vi "运维调试_CODCr.vi"() -> ()   [LabVIEW 2016, in "CODCr库.lvlib"]
uses:
  <vilib>/Utility/miscctls.llb/LVPointTypeDef.ctl
  <vilib>/Plasmionique/MB Master/MB_Master_Serial/MB_Master_Serial.lvclass
  D:/Program Files (x86)/National Instruments/LabVIEW 2016/vi.lib/Plasmionique/MB Master/MB_Master/MB_Master.lvclass
  <vilib>/Plasmionique/MB Master/MB Master.lvlib
  <vilib>/ptbypt/NI_PtbyPt.lvlib
panel:
  out "COM口":string
  in  "空白测试":bool
  in  "隐藏按钮":bool
  in  "写入消解温度时长":bool
  in  "保存KB值":bool
  out "source":string
  in  "标样核查":bool
  out "启动时间":timestamp format="%<%Y/%m/%d %H:%M:%S>T"
  out "主循环次数":i32
  out "status":bool
  out "启动测量模式":T1(ring)
  out "曲线斜率B":sgl format="%#_10g"
  out "曲线斜率K":sgl format="%#_10g"
  out "量程上限":sgl
  out "量程下限":sgl
  out "消解时长":u16
  out "消解温度":u16
  out "测量精度":u16
  out "测量结果":sgl
  out "标样参考值":sgl
  out "量程":u16
  out "工作状态":T1(ring)
  out "仪器时间":timestamp format="%<%X\n%x>T"
  out "关键参数区":T2
  out "状态告警区":T3
  out "测量数据区":T4 {"单位" items=["ug/L", "mg/L", "ppm", "mg/m3", "cm", "ppb", "ug/m3", "%", "nmol/mol", "umol/mol", "MPN/L", "MPN/100ml", "ng/m3", "NTU", "无量纲", "ms/cm", "us/cm", "℃", "mV", "万个/L"]}
  out "系统时间":timestamp format="%<%Y/%m/%d %H:%M:%S>T"
  in  "VISA Resource":refnum<visa-resource-name>="COM9"
  out "Registers":u16[](array[numeric])
  in  "枚举":enum16{"读取", "写入", "读取参数"}(ring)
  in  "停止":bool
  in  "校时":bool
  in  "标样校准":bool
  in  "空白校准":bool
  in  "零点核查":bool
  in  "跨度核查":bool
  in  "水样测试":bool
  in  "返回":bool
  in  "设置":bool
  # "mg/L"
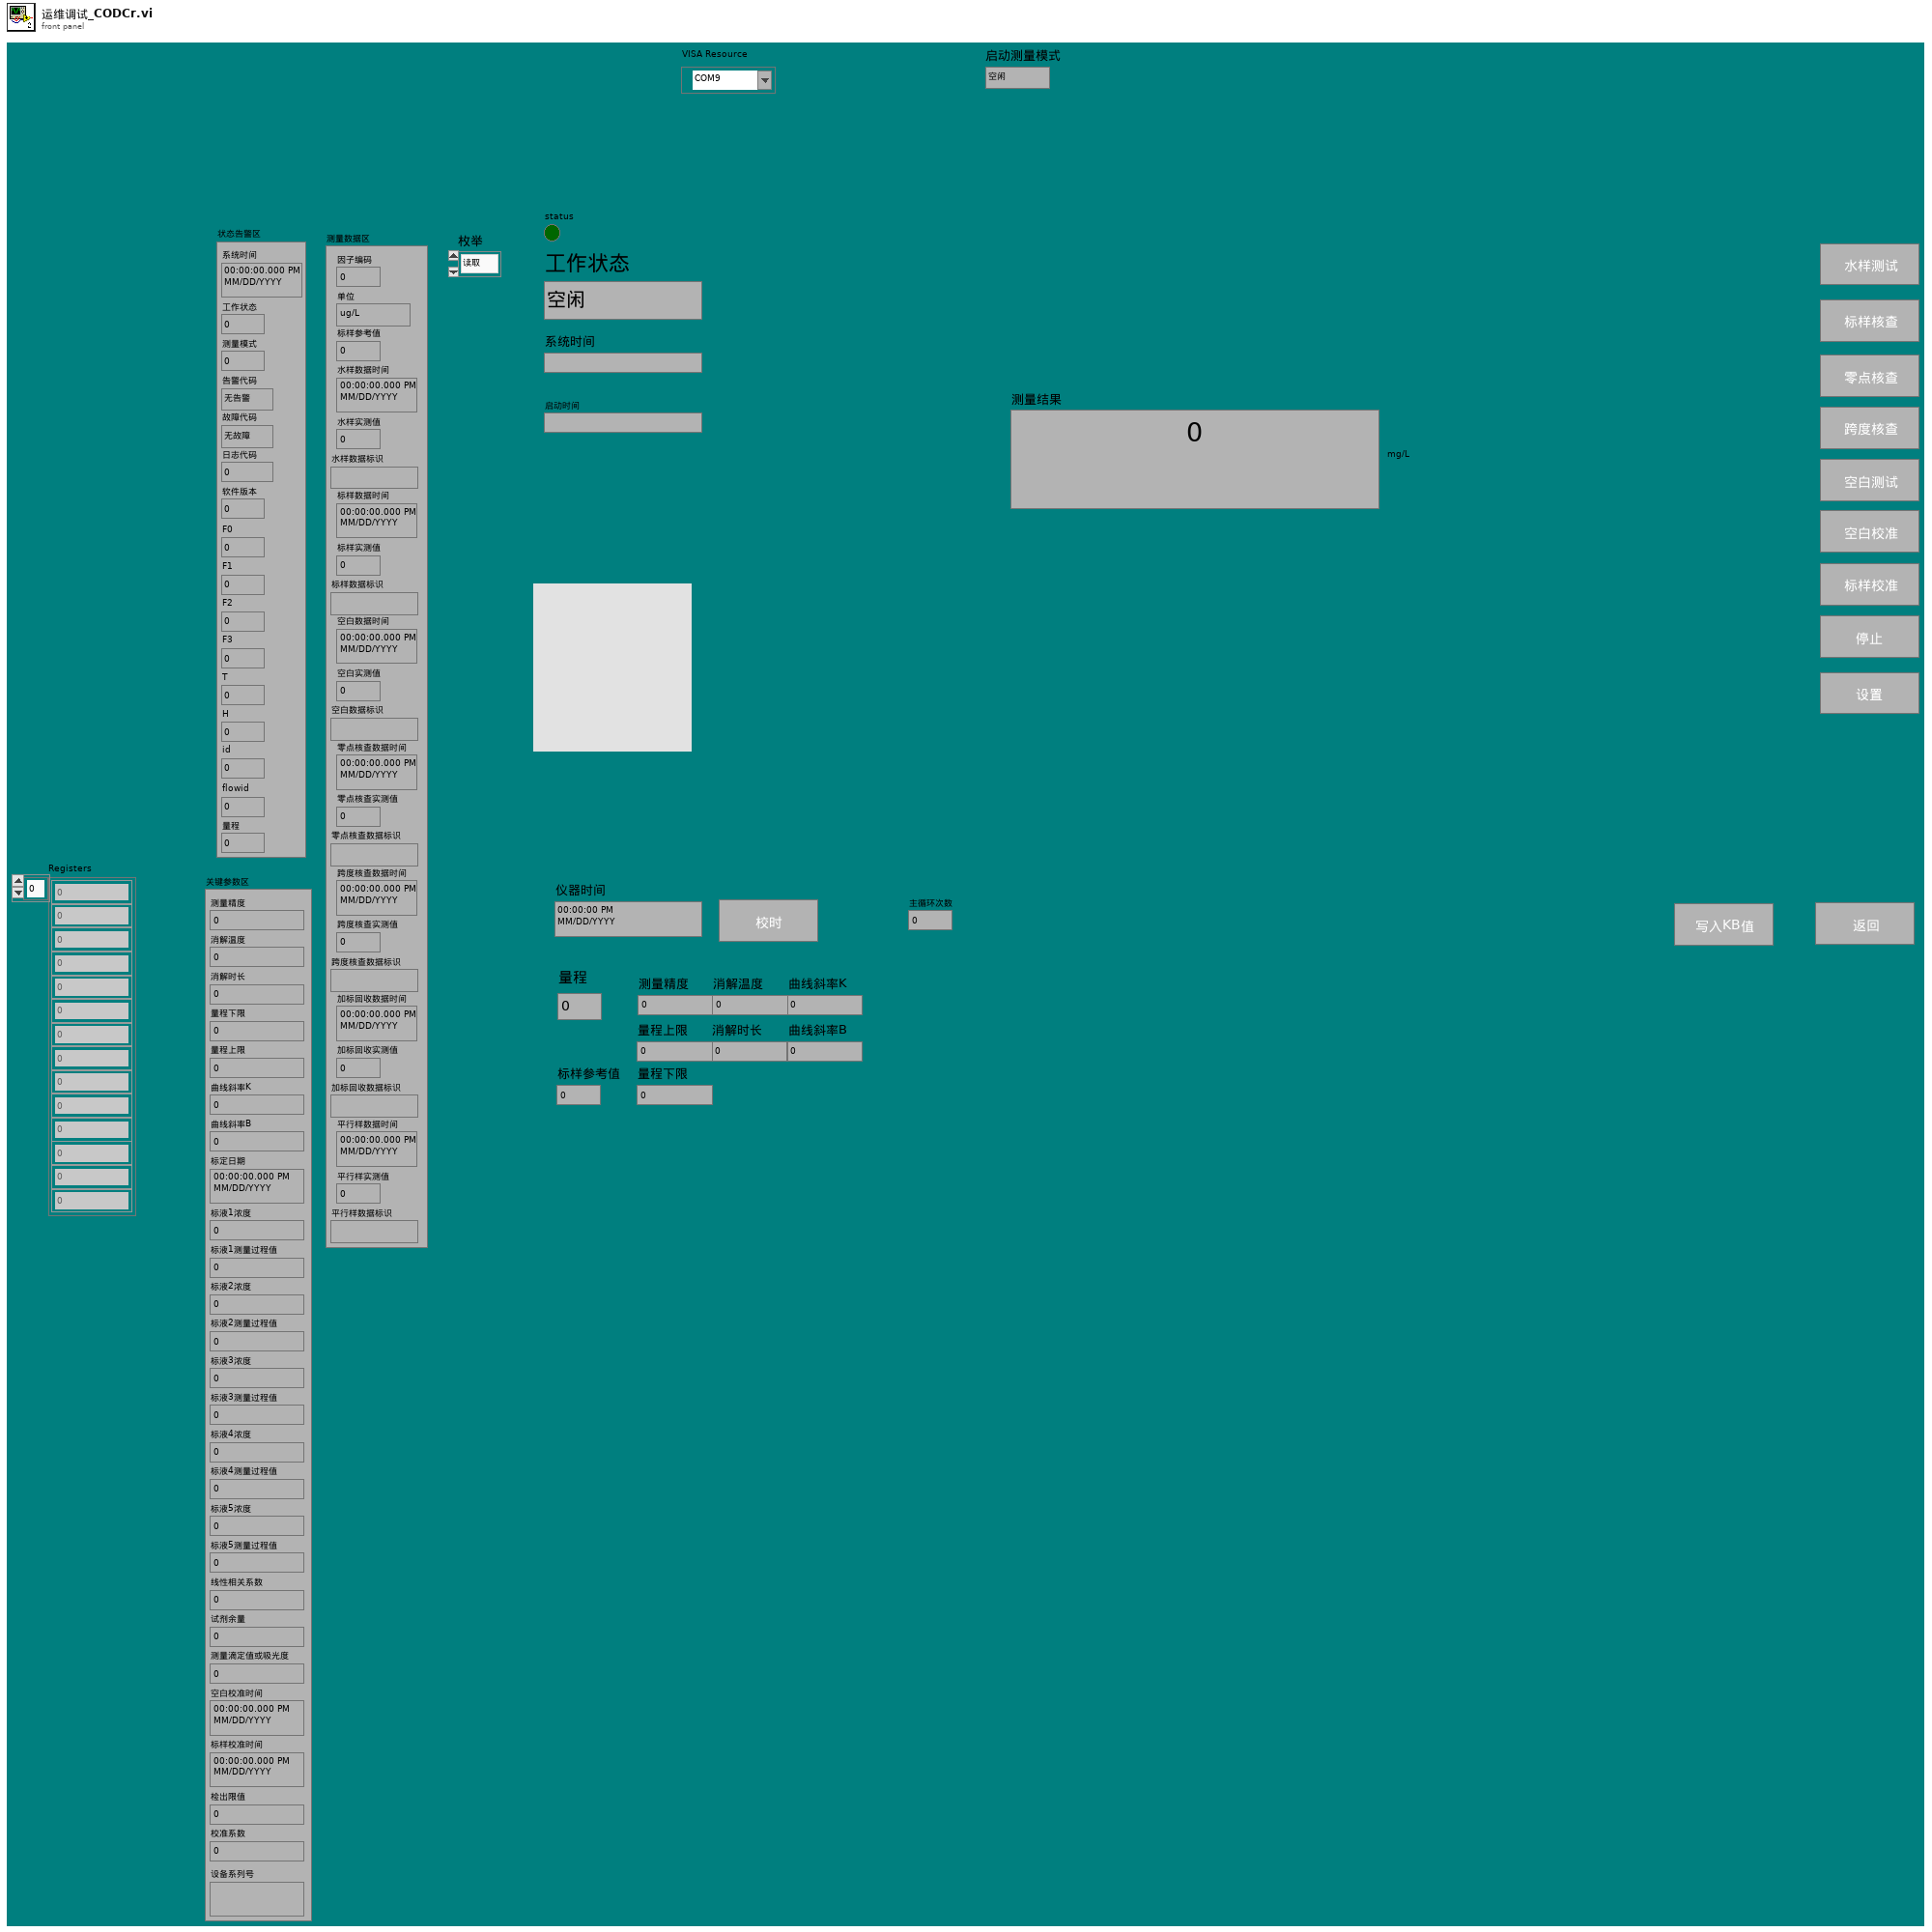
[diagram p1: front panel]
types:
  T1 = enum16{"空闲", "水样测试", "标样核查", "零点核查", "跨度核查", "空白测试", "平行样测试", "加标回收", "空白校准", "标样校准", "初始化（清洗）"}
  T2 = cluster{"测量精度":u16, "消解温度":u16, "消解时长":u16, "量程下限":sgl, "量程上限":sgl, "曲线斜率K":sgl, "曲线斜率B":sgl, "标定日期":timestamp, "标液1浓度":sgl, "标液1测量过程值":sgl, "标液2浓度":sgl, "标液2测量过程值":sgl, "标液3浓度":sgl, "标液3测量过程值":sgl, "标液4浓度":sgl, "标液4测量过程值":sgl, "标液5浓度":sgl, "标液5测量过程值":sgl, "线性相关系数":sgl, "试剂余量":u32, "测量滴定值或吸光度":sgl, "空白校准时间":timestamp, "标样校准时间":timestamp, "检出限值":sgl, "校准系数":sgl, "设备系列号":string}
  T3 = cluster{"系统时间":timestamp, "工作状态":u16, "测量模式":u16, "告警代码":enum16{"无告警", "缺试剂告警", "缺水样告警", "缺蒸馏水告警", "缺标液告警", "仪表漏液告警", "标定异常告警", "超量程告警", "加热异常", "低试剂预警", "超上限告警", "超下限告警", "仪表内部其他异常", "滴定异常告警", "电极异常告警", "量程切换告警", "参数设置告警", "PH电极电位异常", "电导率电极异常", "浊度光度异常", "溶解氧电极异常", "溶解氧光强异常", "温度异常告警", "PH异常告警", "溶解氧异常告警", "电导率异常告警", "浊度异常告警", "叶绿素异常告警", "藻密度异常告警", "蓝绿藻异常告警", "ORP异常告警", "氨氮异常告警", "清洁刷异常告警", "SD卡异常告警", "蓝牙异常告警", "Wifi异常告警", "流程异常告警"}, "故障代码":enum16{"无故障", "电机故障", "温度故障", "通讯故障", "滴定故障"}, "日志代码":u16, "软件版本":u16, "F0":sgl, "F1":sgl, "F2":sgl, "F3":sgl, "T":sgl, "H":sgl, "id":u16, "flowid":u16, "量程":u16}
  T4 = cluster{"因子编码":u32, "单位":u16, "标样参考值":sgl, "水样数据时间":timestamp, "水样实测值":sgl, "水样数据标识":string, "标样数据时间":timestamp, "标样实测值":sgl, "标样数据标识":string, "空白数据时间":timestamp, "空白实测值":sgl, "空白数据标识":string, "零点核查数据时间":timestamp, "零点核查实测值":sgl, "零点核查数据标识":string, "跨度核查数据时间":timestamp, "跨度核查实测值":sgl, "跨度核查数据标识":string, "加标回收数据时间":timestamp, "加标回收实测值":sgl, "加标回收数据标识":string, "平行样数据时间":timestamp, "平行样实测值":sgl, "平行样数据标识":string}
  T5 = cluster{"baud rate (bps)":u32, "stop bits":u16, "parity":u16, "flow control":u16, "timeout":u32, "retries":i32}
  T6 = cluster{"starting address":u16, "number of holding registers":u16}
  T7 = typedef "LVPointTypeDef.ctl" = cluster{"Horizontal":i16, "Vertical":i16}
  T8 = cluster{"运行模式":enum16{"维护模式", "常规模式", "应急模式", "质控模式"}}
  T9 = cluster{"时间标识":timestamp, "监测值":sgl, "单位":u16, "数据标识":string, "因子编码":u32, "标样参考值":sgl, "F0":sgl, "F1":sgl, "F2":sgl, "F3":sgl, "温度":sgl, "湿度":sgl, "量程标识":string}
  T10 = cluster{"系统时间":timestamp, "工作状态":enum16{"空闲", "水样测试", "标样核查", "零点核查", "跨度核查", "空白测试", "平行样测试", "加标回收", "空白校准", "标样校准", "初始化（清洗）"}, "测量模式":enum16{"待机", "连续模式", "周期模式", "定点模式", "受控模式", "手动模式"}, "告警代码":enum16{"无告警", "缺试剂告警", "缺水样告警", "缺蒸馏水告警", "缺标液告警", "仪表漏液告警", "标定异常告警", "超量程告警", "加热异常", "低试剂预警", "超上限告警", "超下限告警", "仪表内部其他异常", "滴定异常告警", "电极异常告警", "量程切换告警", "参数设置告警", "PH电极电位异常", "电导率电极异常", "浊度光度异常", "溶解氧电极异常", "溶解氧光强异常", "温度异常告警", "PH异常告警", "溶解氧异常告警", "电导率异常告警", "浊度异常告警", "叶绿素异常告警", "藻密度异常告警", "蓝绿藻异常告警", "ORP异常告警", "氨氮异常告警", "清洁刷异常告警", "SD卡异常告警", "蓝牙异常告警", "Wifi异常告警", "流程异常告警"}, "故障代码":enum16{"无故障", "电机故障", "温度故障", "通讯故障", "滴定故障"}, "日志代码":u16, "软件版本":u16, "F0":sgl, "F1":sgl, "F2":sgl, "F3":sgl, "T":sgl, "H":sgl, "id":u16, "flowid":u16, "量程":u16}
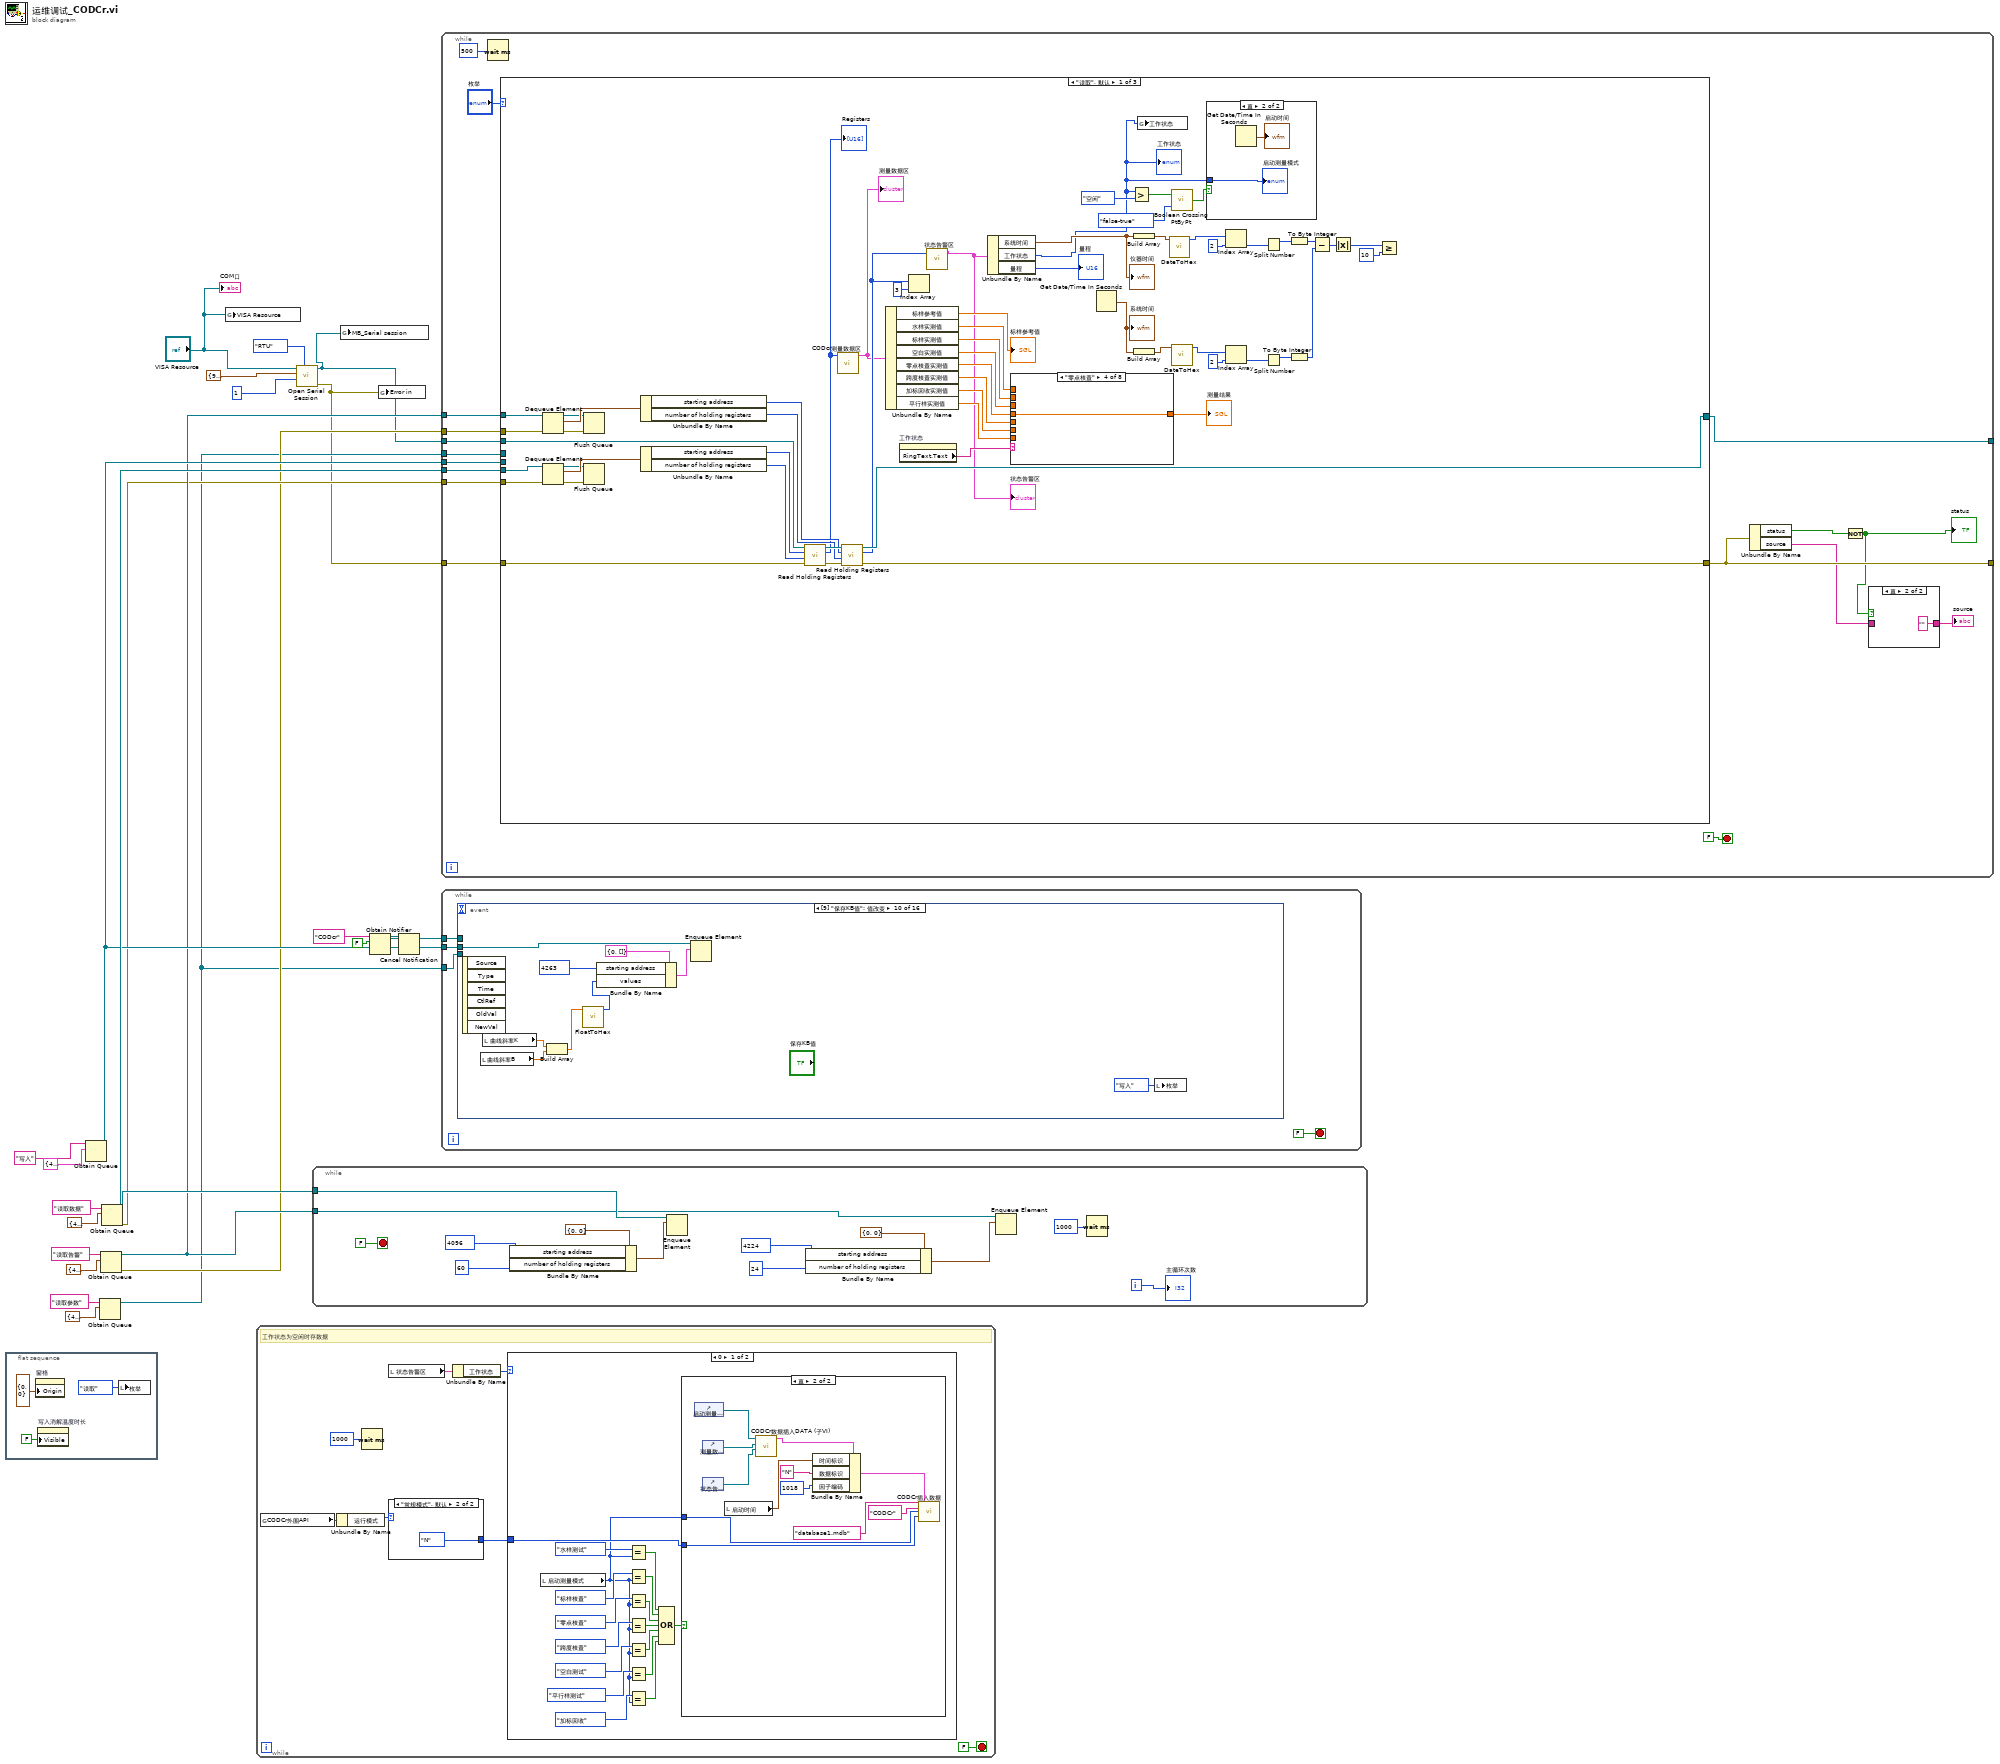
[diagram p0: block diagram]
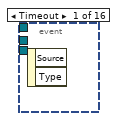
[diagram p2: hidden frame]
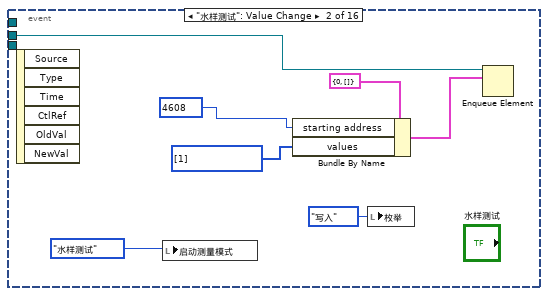
[diagram p3: hidden frame]
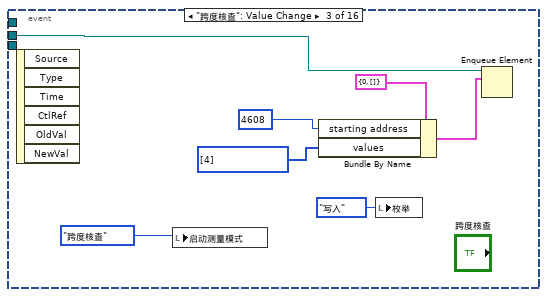
[diagram p4: hidden frame]
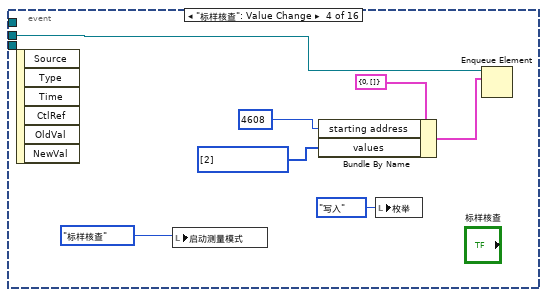
[diagram p5: hidden frame]
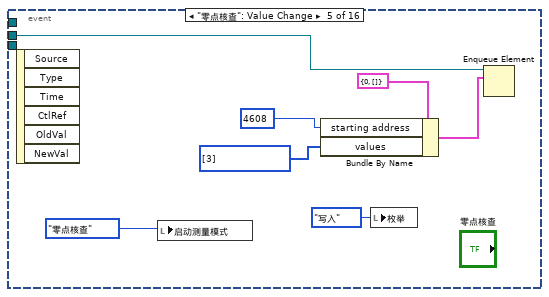
[diagram p6: hidden frame]
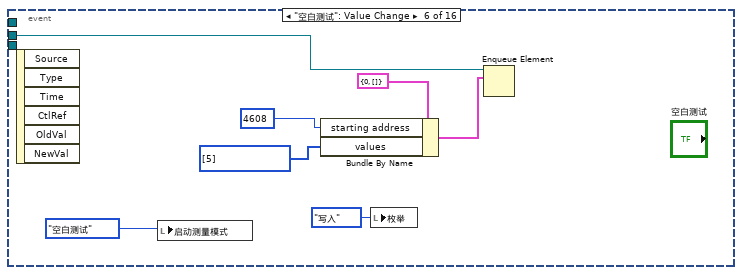
[diagram p7: hidden frame]
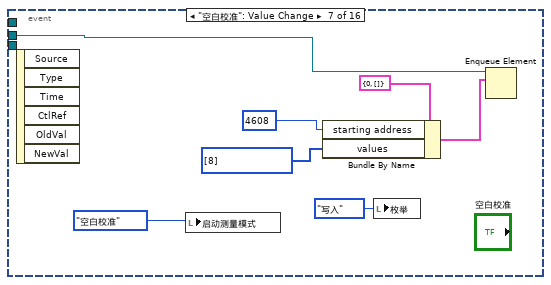
[diagram p8: hidden frame]
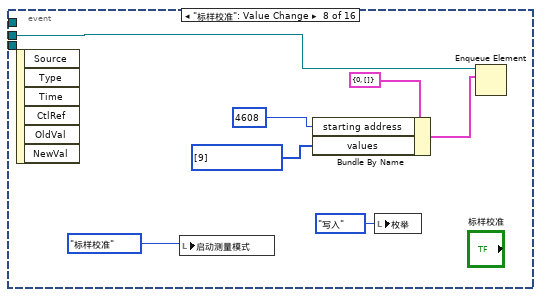
[diagram p9: hidden frame]
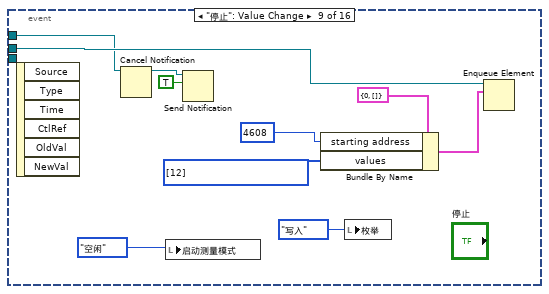
[diagram p10: hidden frame]
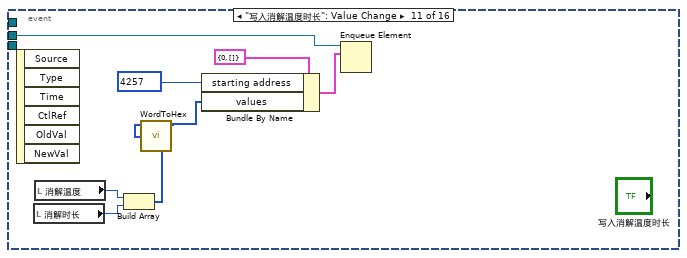
[diagram p11: hidden frame]
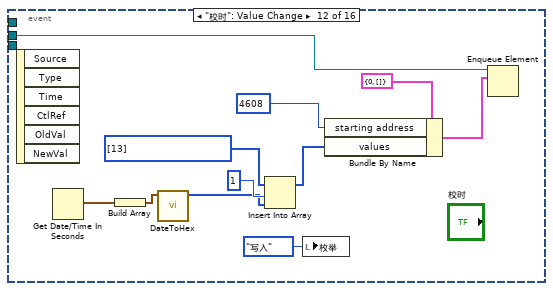
[diagram p12: hidden frame]
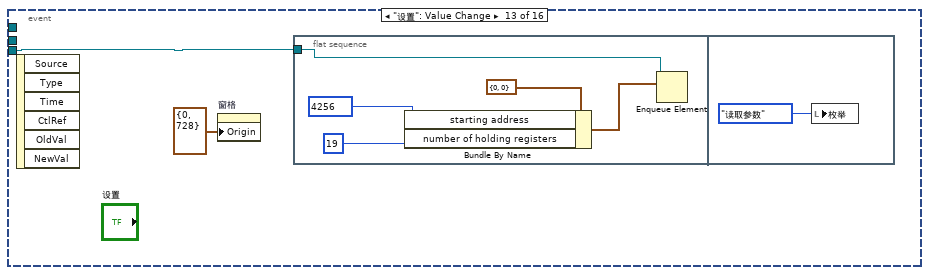
[diagram p13: hidden frame]
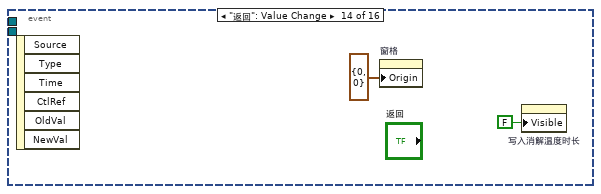
[diagram p14: hidden frame]
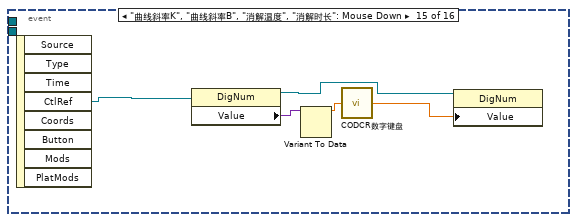
[diagram p15: hidden frame]
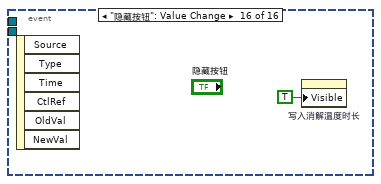
[diagram p16: hidden frame]
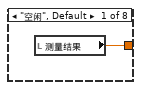
[diagram p18: hidden frame]
diagram:
  n1 = flat-sequence {
    frame #0 {
      n2 = property on="窗格" class="Pane"("Origin"=T7 {"Horizontal"=0, "Vertical"=0} ("原点")) -> ()  [unwired: 2 in, 2 out]
      n3 = property on="写入消解温度时长" class="Bool"("Visible"=FALSE ("可见")) -> ()  [unwired: 2 in, 2 out]
      n4 = local write "枚举"(enum16{"读取", "写入", "读取参数"}."读取" ("枚举")) -> ()
    }
  }
  n5 = Obtain Queue(name (unnamed)="写入" ("名称（未命名）"), element data type=cluster{"starting address":u16, "values":u16[]} {"starting address"=4096, "values"=[]}) -> (queue out=w16:refnum<queue>)  [unwired: 3 in, 2 out]
  n6 = Obtain Queue(name (unnamed)="读取参数" ("名称（未命名）"), element data type=T6 {"starting address"=4096, "number of holding registers"=100}) -> (queue out=w4:refnum<queue>)  [unwired: 3 in, 2 out]
  n7 = Obtain Queue(name (unnamed)="读取告警" ("名称（未命名）"), element data type=T6 {"starting address"=4096, "number of holding registers"=100}) -> (queue out=w13:refnum<queue>, error out=w9:errorcluster)  [unwired: 3 in, 1 out]
  n8 = Obtain Queue(name (unnamed)="读取数据" ("名称（未命名）"), element data type=T6 {"starting address"=4096, "number of holding registers"=100}) -> (queue out=w17:refnum<queue>, error out=w10:errorcluster)  [unwired: 3 in, 1 out]
  n9 = global write "CODcr全局变量.vi" "VISA Resource"("VISA Resource") -> ()
  n10 = while "While循环" {
    stop <- FALSE stop-if-true
    # "工作状态为空闲时存数据"
    n11 = global read "CODCr外部API.vi" "CODCr外围API"() -> (w29:T8)
    n12 = Unbundle By Name(w29) -> ("运行模式"=w28:enum16{"维护模式", "常规模式", "应急模式", "质控模式"})
    n13 = Wait (ms)(milliseconds to wait=u32 1000 ("等待时间（毫秒）")) -> ()  [unwired: 1 out]
    n14 = local read "状态告警区"() -> (w32:T3)
    n15 = case shown="\"常规模式\", 默认" w28 {
      tunnel: [enum16{"N", "M"}."M" ("数据类型") enum16{"N", "M"}."N" ("数据类型")] -> w30
      frame "维护模式" {
      }
      frame "常规模式", Default {
      }
    }
    n16 = Unbundle By Name(w32) -> ("工作状态"=w31:u16)
    n17 = case shown="0" w31 {
      tunnel: w30 -> [w53 _]
      frame 0 {
        n18 = local read "启动测量模式"() -> (w45:T1)
        n19 = Equal?(x=T1."水样测试" ("启动测量模式"), y=w45) -> (x = y?=w44:bool)
        n20 = Equal?(x=T1."标样核查" ("启动测量模式"), y=w45) -> (x = y?=w43:bool)
        n21 = Equal?(x=T1."零点核查" ("启动测量模式"), y=w45) -> (x = y?=w42:bool)
        n22 = Equal?(x=T1."跨度核查" ("启动测量模式"), y=w45) -> (x = y?=w41:bool)
        n23 = Equal?(x=T1."空白测试" ("启动测量模式"), y=w45) -> (x = y?=w40:bool)
        n24 = Equal?(x=T1."平行样测试" ("启动测量模式"), y=w45) -> (x = y?=w39:bool)
        n25 = Equal?(x=T1."加标回收" ("启动测量模式"), y=w45) -> (x = y?=w38:bool)
        n26 = Compound Arithmetic op=OR(w44, w43, w42, w41, w40, w39, w38) -> (w37:bool)
        n27 = case shown="真" w37 {
          tunnel: w45 -> [_ w55]
          tunnel: w53 -> [_ w54]
          frame False {
          }
          frame True {
            n28 = control-ref of="启动测量模式"() -> (w62:refnum<vi>)
            n29 = control-ref of="测量数据区"() -> (w61:refnum<vi>)
            n30 = control-ref of="状态告警区"() -> (w60:refnum<vi>)
            n31 = local read "启动时间"() -> (w65:timestamp)
            n32 = call "CODCr数据插入DATA (子VI).vi"("reference 2"=w60, "reference"=w61, "Enum输入"=w62) -> ("data"=w59:T9)  [unwired: 8 in]
            n33 = Bundle By Name(cluster=w59, "时间标识"=w65, "数据标识"="N", "因子编码"=u32 1018) -> (w58:T9)
            n34 = call "CODCr插入数据.vi"("database"="database1.mdb", "data"=w58, "table"="CODCr", "测量模式"=w55, "数据类型"=w54) -> ()  [unwired: 10 in, 1 out]
          }
        }
      }
      frame 1, Default {
      }
    }
  }
  n35 = call <vilib>:"Open Serial Session.vi"("Mode (RTU)"=enum16{"RTU", "ASCII"}."RTU", "Slave ID"=u8 1, "Serial Config"=T5 {"baud rate (bps)"=9600, "stop bits"=10, "parity"=0, "flow control"=0, "timeout"=1000, "retries"=1}, "VISA Resource"="VISA Resource") -> ("Error out"=w1:errorcluster, "MB_Serial session"=w2:refnum<class "MB_Master_Serial.lvclass">)  [unwired: 6 in]
  n36 = while {
    tunnel: w17 -> [w76]
    tunnel: w13 -> [w67]
    i -> [w66]
    stop <- FALSE stop-if-true
    n37 = Bundle By Name(cluster=T6 {"starting address"=0, "number of holding registers"=0} ("元素"), "starting address"=u16 4096, "number of holding registers"=u16 60) -> (w74:T6)
    n38 = Enqueue Element(queue=w76, element=w74) -> ()  [unwired: 2 in, 3 out]
    n39 = Bundle By Name(cluster=T6 {"starting address"=0, "number of holding registers"=0} ("元素"), "starting address"=u16 4224, "number of holding registers"=u16 24) -> (w68:T6)
    n40 = Enqueue Element(queue=w67, element=w68) -> ()  [unwired: 2 in, 3 out]
    n41 = Wait (ms)(milliseconds to wait=u32 1000 ("等待时间（毫秒）")) -> ()  [unwired: 1 out]
    "主循环次数" <- w66
  }
  n42 = global write "CODcr全局变量.vi" "MB_Serial session"(w2) -> ()
  n43 = Obtain Notifier(name (unnamed)="CODcr" ("名称（未命名）"), notification data type=FALSE) -> (notifier out=w5:refnum<notifier>)  [unwired: 2 in, 2 out]
  n44 = global write "CODcr全局变量.vi" "Error in"(w1) -> ()
  n45 = Cancel Notification(0:w5) -> (8:w6:refnum<notifier>)  [unwired: 1 in, 2 out]
  n46 = while {
    tunnel: w16 -> [w92]
    tunnel: w17 -> [w91]
    tunnel: w13 -> [w90]
    tunnel: w4 -> [w89]
    tunnel: w10 -> [w87]
    tunnel: w9 -> [w86]
    tunnel: w1 -> [w85]
    tunnel: [w83] -> _
    tunnel: w2 -> [w93]
    tunnel: [w88] -> _
    stop <- FALSE stop-if-true
    n47 = Wait (ms)(milliseconds to wait=u32 500 ("等待时间（毫秒）")) -> ()  [unwired: 1 out]
    n48 = case shown="\"读取\", 默认" "枚举" {
      tunnel: w93 -> [w155 w172 w195]
      tunnel: w85 -> [w133 w171 w194]
      tunnel: w92 -> [_ w170 _]
      tunnel: w91 -> [w154 _ _]
      tunnel: w90 -> [w150 _ _]
      tunnel: w89 -> [_ _ w196]
      tunnel: [w132 w166 w184] -> w83
      tunnel: [w118 w167 w185] -> w88
      tunnel: w87 -> [w112 _ _]
      tunnel: w86 -> [w109 _ _]
      frame "读取", Default {
        n49 = Dequeue Element(queue=w150, error in (no error)=w109) -> (queue out=w111:refnum<queue>, element=w149:T6, error out=w110:errorcluster)  [unwired: 1 in, 1 out]
        n50 = Dequeue Element(queue=w154, error in (no error)=w112) -> (queue out=w114:refnum<queue>, element=w153:T6, error out=w113:errorcluster)  [unwired: 1 in, 1 out]
        n51 = Flush Queue(queue=w111, error in (no error)=w110) -> ()  [unwired: 3 out]
        n52 = Flush Queue(queue=w114, error in (no error)=w113) -> ()  [unwired: 3 out]
        n53 = Unbundle By Name(w149) -> ("starting address"=w146:u16, "number of holding registers"=w145:u16)
        n54 = Unbundle By Name(w153) -> ("starting address"=w152:u16, "number of holding registers"=w151:u16)
        n55 = call <vilib>:"Read Holding Registers.vi"("error in (no error)"=w133, "quantity"=w151, "starting address"=w152, "MB session in"=w155) -> ("error out"=w147:errorcluster, "Registers"=w102:u16[], "MB session out"=w148:refnum<class "MB_Master_Serial.lvclass">)  [unwired: 5 in]
        "Registers" <- w102
        n56 = call "CODcr测量数据区.vi"("数组"=w102) -> ("测量数据区"=w103:T4)  [unwired: 10 in]
        "测量数据区" <- w103
        n57 = call <vilib>:"Read Holding Registers.vi"("error in (no error)"=w147, "quantity"=w145, "starting address"=w146, "MB session in"=w148) -> ("error out"=w132:errorcluster, "Registers"=w106:u16[], "MB session out"=w118:refnum<class "MB_Master_Serial.lvclass">)  [unwired: 5 in]
        n58 = Unbundle By Name(w103) -> ("标样参考值"=→"标样参考值":sgl, "水样实测值"=w141:sgl, "标样实测值"=w139:sgl, "空白实测值"=w136:sgl, "零点核查实测值"=w138:sgl, "跨度核查实测值"=w137:sgl, "加标回收实测值"=w134:sgl, "平行样实测值"=w135:sgl)
        n59 = property on="工作状态" class="Enum (严格)"() -> ("RingText.Text"=w142:string)  [unwired: 2 in, 2 out]
        n60 = Index Array(array=w106, index=3 ("索引")) -> ()  [unwired: 1 out]
        n61 = call "状态告警区.vi"("数组"=w106) -> ("状态告警区"=w105:T10)  [unwired: 10 in]
        "状态告警区" <- w105
        n62 = Unbundle By Name(w105) -> ("系统时间"=w119:timestamp, "工作状态"=w104:T1, "量程"=→"量程":u16)
        "仪器时间" <- w119
        "工作状态" <- w104
        n63 = case shown="\"零点核查\"" w142 {
          tunnel: w141 -> [_ w157 _ _ _ _ _ _]
          tunnel: [w156 w157 w158 w159 w160 w161 w162 w163] -> w140
          tunnel: w139 -> [_ _ w158 _ _ _ _ _]
          tunnel: w138 -> [_ _ _ w159 _ _ _ _]
          tunnel: w137 -> [_ _ _ _ w160 _ _ _]
          tunnel: w136 -> [_ _ _ _ _ w161 _ _]
          tunnel: w135 -> [_ _ _ _ _ _ w162 _]
          tunnel: w134 -> [_ _ _ _ _ _ _ w163]
          frame "空闲", Default {
            n64 = local read "测量结果"() -> (w156:sgl)
          }
          frame "水样测试" {
          }
          frame "标样核查" {
          }
          frame "零点核查" {
          }
          frame "跨度核查" {
          }
          frame "空白测试" {
          }
          frame "平行样测试" {
          }
          frame "加标回收" {
          }
        }
        "测量结果" <- w140
        n65 = Get Date/Time In Seconds() -> (seconds since 1Jan1904=w120:timestamp)
        "系统时间" <- w120
        n66 = Greater?(x=w104, y=T1."空闲") -> (0:w117:bool)
        n67 = Build Array(w119) -> (w100:timestamp[])
        n68 = Build Array(w120) -> (w101:timestamp[])
        n69 = global write "CODCr工作状态.vi" "工作状态"(w104) -> ()
        n70 = call "DateToHex.vi"("DATE"=w100) -> ("数组"=w99:u16[])  [unwired: 10 in]
        n71 = call <vilib>:"Boolean Crossing PtByPt.vi"("direction"=enum16{"either", "false-true", "true-false"}."false-true", "input"=w117) -> ("crossing"=w116:bool)  [unwired: 1 in]
        n72 = call "DateToHex.vi"("DATE"=w101) -> ("数组"=w98:u16[])  [unwired: 10 in]
        n73 = case shown="真" w116 {
          tunnel: w104 -> [_ w164]
          frame False {
          }
          frame True {
            n74 = Get Date/Time In Seconds() -> (seconds since 1Jan1904=→"启动时间":timestamp)
            "启动测量模式" <- w164
          }
        }
        n75 = Index Array(array=w99, index=2 ("索引")) -> (element=w123:u16)
        n76 = Index Array(array=w98, index=2 ("索引")) -> (element=w122:u16)
        n77 = Split Number(x=w123) -> (hi(x)=w128:u8)  [unwired: 1 out]
        n78 = Split Number(x=w122) -> (hi(x)=w125:u8)  [unwired: 1 out]
        n79 = To Byte Integer(number=w128) -> (8bit integer=w129:i8)
        n80 = To Byte Integer(number=w125) -> (8bit integer=w126:i8)
        n81 = Subtract(x=w129, y=w126) -> (x-y=w127:i8)
        n82 = Absolute Value(x=w127) -> (abs(x)=w130:i8)
        n83 = Greater Or Equal?(x=w130, y=i8 10) -> ()  [unwired: 1 out]
      }
      frame "写入" {
        n84 = flat-sequence {
          tunnel: w172 -> [w180]
          tunnel: w171 -> [w179]
          tunnel: w170 -> [w176]
          tunnel: [w178] -> w169
          tunnel: [w177] -> w168
          tunnel: w169 -> [w182]
          tunnel: w168 -> [w181]
          tunnel: [w182] -> w167
          tunnel: [w181] -> w166
          frame #0 {
            n85 = Dequeue Element(queue=w176) -> (element=w175:cluster{"starting address":u16, "values":u16[]})  [unwired: 2 in, 3 out]
            n86 = Unbundle By Name(w175) -> ("starting address"=w174:u16, "values"=w173:u16[])
            n87 = call <vilib>:"Write Multiple Registers.vi"("error in (no error)"=w179, "values"=w173, "starting address"=w174, "MB session in"=w180) -> ("error out"=w177:errorcluster, "MB session out"=w178:refnum<class "MB_Master_Serial.lvclass">)  [unwired: 6 in]
          }
          frame #1 {
            n88 = local write "枚举"(enum16{"读取", "写入", "读取参数"}."读取" ("枚举")) -> ()
          }
        }
      }
      frame "读取参数" {
        n89 = local write "枚举"(enum16{"读取", "写入", "读取参数"}."读取" ("枚举")) -> ()
        n90 = Dequeue Element(queue=w196, timeout in ms (-1)=1000 ("超时毫秒(-1)")) -> (element=w203:T6)  [unwired: 1 in, 3 out]
        n91 = Unbundle By Name(w203) -> ("starting address"=w202:u16, "number of holding registers"=w201:u16)
        n92 = call <vilib>:"Read Holding Registers.vi"("error in (no error)"=w194, "quantity"=w201, "starting address"=w202, "MB session in"=w195) -> ("error out"=w198:errorcluster, "Registers"=w200:u16[], "MB session out"=w185:refnum<class "MB_Master_Serial.lvclass">)  [unwired: 5 in]
        n93 = call "关键参数区.vi"("数组"=w200) -> ("关键参数区"=w197:T2)  [unwired: 10 in]
        "关键参数区" <- w197
        n94 = Unbundle By Name(w197) -> ("测量精度"=→"测量精度":u16, "消解温度"=→"消解温度":u16, "消解时长"=→"消解时长":u16, "量程下限"=→"量程下限":sgl, "量程上限"=→"量程上限":sgl, "曲线斜率K"=→"曲线斜率K":sgl, "曲线斜率B"=→"曲线斜率B":sgl)
        n95 = call <vilib>:"Clear Errors.vi"("error in (no error)"=w198) -> ("error out"=w184:errorcluster)  [unwired: 5 in, 1 out]
      }
    }
    n96 = Unbundle By Name(w83) -> ("status"=w84:bool, "source"=w81:string)
    n97 = Not(x=w84) -> (.not. x?=w80:bool)
    "status" <- w80
    n98 = case shown="真" w80 {
      tunnel: w81 -> [w96 _]
      tunnel: [w96 "" ("source")] -> w79
      frame False {
      }
      frame True {
      }
    }
    "source" <- w79
  }
  n99 = while {
    tunnel: w16 -> [w206]
    tunnel: w6 -> [w205]
    tunnel: w4 -> [w204]
    stop <- FALSE stop-if-true
    n100 = event shown="[9] \"保存KB值\": 值改变" {
      selector: _ -> [_ _ _ _ _ _ _ _ _ _ _ _ _ _ _ _]
      dyn-events: _ -> [_ _ _ _ _ _ _ _ _ _ _ _ _ _ _ _]
      timeout: _ -> [_ _ _ _ _ _ _ _ _ _ _ _ _ _ _ _]
      tunnel: w206 -> [_ w214 w217 w224 w231 w238 w245 w252 w262 w274 w280 w291 _ _ _ _]
      tunnel: w205 -> [_ _ _ _ _ _ _ _ w260 _ _ _ _ _ _ _]
      tunnel: w204 -> [_ _ _ _ _ _ _ _ _ _ _ _ w295 _ _ _]
      event Timeout {
        n101 = event-data() -> ()  [unwired: 1 in, 2 out]
      }
      event "水样测试": Value Change {
        n102 = event-data() -> ()  [unwired: 1 in, 6 out]
        n103 = local write "启动测量模式"(T1."水样测试" ("启动测量模式")) -> ()
        n104 = Bundle By Name(cluster=cluster{"starting address":u16, "values":u16[]} {"starting address"=0, "values"=[]} ("元素"), "starting address"=u16 4608, "values"=u16[] [1]) -> (w212:cluster{"starting address":u16, "values":u16[]})
        n105 = local write "枚举"(enum16{"读取", "写入", "读取参数"}."写入" ("枚举")) -> ()
        n106 = Enqueue Element(queue=w214, element=w212) -> ()  [unwired: 2 in, 3 out]
      }
      event "跨度核查": Value Change {
        n107 = event-data() -> ()  [unwired: 1 in, 6 out]
        n108 = local write "启动测量模式"(T1."跨度核查" ("启动测量模式")) -> ()
        n109 = Bundle By Name(cluster=cluster{"starting address":u16, "values":u16[]} {"starting address"=0, "values"=[]} ("元素"), "starting address"=u16 4608, "values"=u16[] [4]) -> (w220:cluster{"starting address":u16, "values":u16[]})
        n110 = local write "枚举"(enum16{"读取", "写入", "读取参数"}."写入" ("枚举")) -> ()
        n111 = Enqueue Element(queue=w217, element=w220) -> ()  [unwired: 2 in, 3 out]
      }
      event "标样核查": Value Change {
        n112 = event-data() -> ()  [unwired: 1 in, 6 out]
        n113 = local write "启动测量模式"(T1."标样核查" ("启动测量模式")) -> ()
        n114 = Bundle By Name(cluster=cluster{"starting address":u16, "values":u16[]} {"starting address"=0, "values"=[]} ("元素"), "starting address"=u16 4608, "values"=u16[] [2]) -> (w227:cluster{"starting address":u16, "values":u16[]})
        n115 = local write "枚举"(enum16{"读取", "写入", "读取参数"}."写入" ("枚举")) -> ()
        n116 = Enqueue Element(queue=w224, element=w227) -> ()  [unwired: 2 in, 3 out]
      }
      event "零点核查": Value Change {
        n117 = event-data() -> ()  [unwired: 1 in, 6 out]
        n118 = local write "启动测量模式"(T1."零点核查" ("启动测量模式")) -> ()
        n119 = Bundle By Name(cluster=cluster{"starting address":u16, "values":u16[]} {"starting address"=0, "values"=[]} ("元素"), "starting address"=u16 4608, "values"=u16[] [3]) -> (w234:cluster{"starting address":u16, "values":u16[]})
        n120 = local write "枚举"(enum16{"读取", "写入", "读取参数"}."写入" ("枚举")) -> ()
        n121 = Enqueue Element(queue=w231, element=w234) -> ()  [unwired: 2 in, 3 out]
      }
      event "空白测试": Value Change {
        n122 = event-data() -> ()  [unwired: 1 in, 6 out]
        n123 = local write "启动测量模式"(T1."空白测试" ("启动测量模式")) -> ()
        n124 = Bundle By Name(cluster=cluster{"starting address":u16, "values":u16[]} {"starting address"=0, "values"=[]} ("元素"), "starting address"=u16 4608, "values"=u16[] [5]) -> (w241:cluster{"starting address":u16, "values":u16[]})
        n125 = local write "枚举"(enum16{"读取", "写入", "读取参数"}."写入" ("枚举")) -> ()
        n126 = Enqueue Element(queue=w238, element=w241) -> ()  [unwired: 2 in, 3 out]
      }
      event "空白校准": Value Change {
        n127 = event-data() -> ()  [unwired: 1 in, 6 out]
        n128 = local write "启动测量模式"(T1."空白校准" ("启动测量模式")) -> ()
        n129 = Bundle By Name(cluster=cluster{"starting address":u16, "values":u16[]} {"starting address"=0, "values"=[]} ("元素"), "starting address"=u16 4608, "values"=u16[] [8]) -> (w248:cluster{"starting address":u16, "values":u16[]})
        n130 = local write "枚举"(enum16{"读取", "写入", "读取参数"}."写入" ("枚举")) -> ()
        n131 = Enqueue Element(queue=w245, element=w248) -> ()  [unwired: 2 in, 3 out]
      }
      event "标样校准": Value Change {
        n132 = event-data() -> ()  [unwired: 1 in, 6 out]
        n133 = local write "启动测量模式"(T1."标样校准" ("启动测量模式")) -> ()
        n134 = Bundle By Name(cluster=cluster{"starting address":u16, "values":u16[]} {"starting address"=0, "values"=[]} ("元素"), "starting address"=u16 4608, "values"=u16[] [9]) -> (w255:cluster{"starting address":u16, "values":u16[]})
        n135 = local write "枚举"(enum16{"读取", "写入", "读取参数"}."写入" ("枚举")) -> ()
        n136 = Enqueue Element(queue=w252, element=w255) -> ()  [unwired: 2 in, 3 out]
      }
      event "停止": Value Change {
        n137 = event-data() -> ()  [unwired: 1 in, 6 out]
        n138 = Cancel Notification(0:w260) -> (8:w259:refnum<notifier>)  [unwired: 1 in, 2 out]
        n139 = local write "启动测量模式"(T1."空闲" ("启动测量模式")) -> ()
        n140 = Send Notification(notification=TRUE ("通知"), notifier=w259) -> ()  [unwired: 1 in, 2 out]
        n141 = Bundle By Name(cluster=cluster{"starting address":u16, "values":u16[]} {"starting address"=0, "values"=[]} ("元素"), "starting address"=u16 4608, "values"=u16[] [12]) -> (w265:cluster{"starting address":u16, "values":u16[]})
        n142 = local write "枚举"(enum16{"读取", "写入", "读取参数"}."写入" ("枚举")) -> ()
        n143 = Enqueue Element(queue=w262, element=w265) -> ()  [unwired: 2 in, 3 out]
      }
      event "保存KB值": Value Change {
        n144 = event-data() -> ()  [unwired: 1 in, 6 out]
        n145 = local read "曲线斜率B"() -> (w269:sgl)
        n146 = local read "曲线斜率K"() -> (w270:sgl)
        n147 = Build Array(w270, w269) -> (w268:sgl[])
        n148 = call "FloatToHex.vi"("浮点数"=w268) -> ("DCBA整形输出"=w267:u16[])  [unwired: 10 in]
        n149 = Bundle By Name(cluster=cluster{"starting address":u16, "values":u16[]} {"starting address"=0, "values"=[]} ("元素"), "starting address"=u16 4263, "values"=w267) -> (w272:cluster{"starting address":u16, "values":u16[]})
        n150 = Enqueue Element(queue=w274, element=w272) -> ()  [unwired: 2 in, 3 out]
        n151 = local write "枚举"(enum16{"读取", "写入", "读取参数"}."写入" ("枚举")) -> ()
      }
      event "写入消解温度时长": Value Change {
        n152 = event-data() -> ()  [unwired: 1 in, 6 out]
        n153 = local read "消解时长"() -> (w278:u16)
        n154 = local read "消解温度"() -> (w279:u16)
        n155 = Build Array(w279, w278) -> (w277:u16[])
        n156 = call "WordToHex.vi"("WORD"=w277) -> ("数组"=w276:u16[])  [unwired: 10 in]
        n157 = Bundle By Name(cluster=cluster{"starting address":u16, "values":u16[]} {"starting address"=0, "values"=[]} ("元素"), "starting address"=u16 4257, "values"=w276) -> (w282:cluster{"starting address":u16, "values":u16[]})
        n158 = Enqueue Element(queue=w280, element=w282) -> ()  [unwired: 2 in, 3 out]
      }
      event "校时": Value Change {
        n159 = event-data() -> ()  [unwired: 1 in, 6 out]
        n160 = Get Date/Time In Seconds() -> (seconds since 1Jan1904=w290:timestamp)
        n161 = Build Array(w290) -> (w285:timestamp[])
        n162 = call "DateToHex.vi"("DATE"=w285) -> ("数组"=w284:u16[])  [unwired: 10 in]
        n163 = Insert Into Array(array=u16[] [13] ("values"), index=1 ("索引"), new element=w284) -> (w287:u16[])
        n164 = local write "枚举"(enum16{"读取", "写入", "读取参数"}."写入" ("枚举")) -> ()
        n165 = Bundle By Name(cluster=cluster{"starting address":u16, "values":u16[]} {"starting address"=0, "values"=[]} ("元素"), "starting address"=u16 4608, "values"=w287) -> (w293:cluster{"starting address":u16, "values":u16[]})
        n166 = Enqueue Element(queue=w291, element=w293) -> ()  [unwired: 2 in, 3 out]
      }
      event "设置": Value Change {
        n167 = event-data() -> ()  [unwired: 1 in, 6 out]
        n168 = property on="窗格" class="Pane"("Origin"=T7 {"Horizontal"=0, "Vertical"=728} ("原点")) -> ()  [unwired: 2 in, 2 out]
        n169 = flat-sequence {
          tunnel: w295 -> [w297]
          frame #0 {
            n170 = Bundle By Name(cluster=T6 {"starting address"=0, "number of holding registers"=0} ("元素"), "starting address"=u16 4256, "number of holding registers"=u16 19) -> (w301:T6)
            n171 = Enqueue Element(queue=w297, element=w301) -> ()  [unwired: 2 in, 3 out]
          }
          frame #1 {
            n172 = local write "枚举"(enum16{"读取", "写入", "读取参数"}."读取参数" ("枚举")) -> ()
          }
        }
      }
      event "返回": Value Change {
        n173 = event-data() -> ()  [unwired: 1 in, 6 out]
        n174 = property on="窗格" class="Pane"("Origin"=T7 {"Horizontal"=0, "Vertical"=0} ("原点")) -> ()  [unwired: 2 in, 2 out]
        n175 = property on="写入消解温度时长" class="Bool"("Visible"=FALSE ("可见")) -> ()  [unwired: 2 in, 2 out]
      }
      event "曲线斜率K", "曲线斜率B", "消解温度", "消解时长": Mouse Down {
        n176 = event-data() -> ("CtlRef"=w307:refnum<vi>)  [unwired: 1 in, 7 out]
        n177 = property class="DigNum"(reference=w307) -> (reference out=w308:refnum<vi>, "Value"=w306:variant)  [unwired: 1 in, 1 out]
        n178 = Variant To Data(Variant=w306) -> (data=w305:sgl)  [unwired: 2 in, 1 out]
        n179 = call "CODCR数字键盘.vi"("OldNumber"=w305) -> ("NewNumber"=w309:sgl)
        n180 = property class="DigNum"(reference=w308, "Value"=w309) -> ()  [unwired: 1 in, 2 out]
      }
      event "隐藏按钮": Value Change {
        n181 = event-data() -> ()  [unwired: 1 in, 6 out]
        n182 = property on="写入消解温度时长" class="Bool"("Visible"=TRUE ("可见")) -> ()  [unwired: 2 in, 2 out]
      }
    }
  }
  "COM口" <- "VISA Resource"
